vi "Measure Base.vi"(0 "eye scan in":refnum<class "niHighSpeedSerial Eye Scan v1 Host.lvclass">, 5 "requested number of new points":i32, 7 "timeout (100 ms)":dbl, 11 "error in":errorcluster) -> (4 "eye scan out":refnum<class "niHighSpeedSerial Eye Scan v1 Host.lvclass">, 6 "retrieved number of new points":i32, 8 "last point measured?":bool, 10 "timed out?":bool, 15 "error out":errorcluster)   [LabVIEW 2014, in "niHighSpeedSerial Eye Scan v1 Host.lvclass"]
doc: "The base Measure VI used by the various Measure VIs. This VI does the actual measurement, while the calling VIs do the data formatting.\n\n<B>Input Parameters</B>\n\n<B>eye scan in</B> Takes in a reference to your session from the previous VI.\n\n<B>requested number of new points</B> The number of new points to return, assuming that timeout is not reached, the entire scan doesn't complete, and no errors occur.\n\n<B>timeout (100 ms)</B> The amount of time (in seconds) before timing timing out.\nSpecifying '-1' prevents 'timed out' from ever returning true.\n\n<B>error in</B> describes error conditions that occur before this node runs. This input provides standard 'error in' functionality.\n\n<B>Output Parameters</B>\n\n<B>eye scan out</B> passes a reference to your session to the next VI.\n\n<B>retrieved number of new points</B> The number of new points that were retrieved in this call to Measure.\n\n<B>last point measured?</B> returns true if Eye Scan has completed measuring all points that it was configured to measure.\n\n<B>timed out?</B> returns true if at least 'timeout' amount of time has passed.\n\n<B>error out</B> contains error information. This output provides standard 'error out' functionality."
uses:
  <instrlib>/niHighSpeedSerial/Eye Scan/v1/Host/Eye Scan/niHighSpeedSerial Eye Scan v1 Host.lvclass
  <instrlib>/niHighSpeedSerial/Eye Scan/v1/Host/Eye Scan/niHighSpeedSerial Eye Scan v1 Host.lvclass/niHighSpeedSerial Eye Scan v1 Host.ctl
  <vilib>/Utility/error.llb/Error Cluster From Error Code.vi
  <vilib>/ErrorRing/Error Ring.xnode
  <instrlib>/niHighSpeedSerial/Eye Scan/v1/Host/Common/niHighSpeedSerial Eye Scan Common v1 Host.lvlib
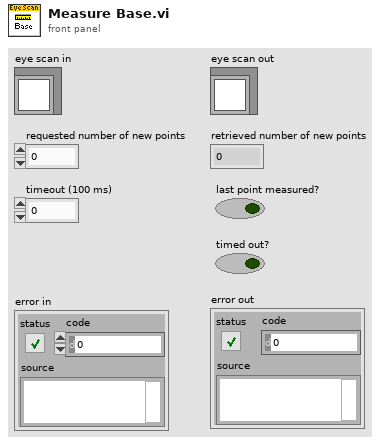
[diagram p1: front panel]
types:
  T1 = typedef "niHighSpeedSerial Eye Scan v1 Host.lvclass/Private Data.ctl" = cluster{"instruction target":refnum<class "niInstr Instruction Target v1 Host.lvclass">, "channels":T2[], "measure state":T3, "rx output divider":T4, "equalization mode":T5, "rx data width":T6, "BER floor":dbl, "number of points completed":i32, "rx output divider configured?":bool, "equalization mode configured?":bool, "rx data width configured?":bool}
  T2 = typedef "niHighSpeedSerial Eye Scan v1 Host.lvclass/Channel Data.ctl" = cluster{"instance":u8, "channel":refnum<class "niHighSpeedSerial Eye Scan Single Point v1 Host.lvclass">, "point iterator":refnum<class "niHighSpeedSerial Eye Scan Point Iterator v1 Host.lvclass">}
  T3 = typedef "niHighSpeedSerial Eye Scan v1 Host.lvclass/Measure State.ctl" = enum16{"Uninitialized", "Initialized", "Ready", "Measuring", "Finished", "Aborted"}
  T4 = typedef "niHighSpeedSerial Eye Scan Common v1 Host.lvlib/RX Output Divider.ctl" = enum16{"1", "2", "4", "8", "16"}
  T5 = typedef "niHighSpeedSerial Eye Scan Common v1 Host.lvlib/Equalization Mode.ctl" = enum16{"DFE", "LPM"}
  T6 = typedef "niHighSpeedSerial Eye Scan Common v1 Host.lvlib/Data Width.ctl" = enum16{"16 Bit", "20 Bit", "32 Bit", "40 Bit"}
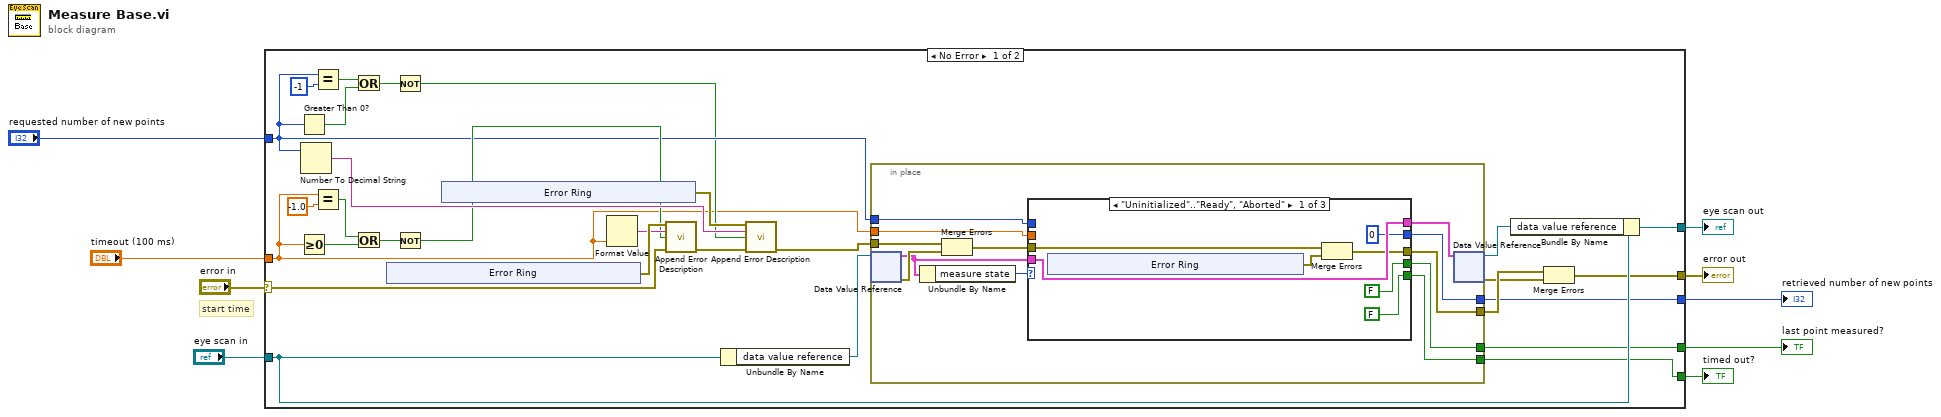
[diagram p0: block diagram]
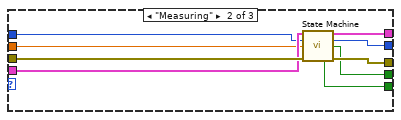
[diagram p2: hidden frame]
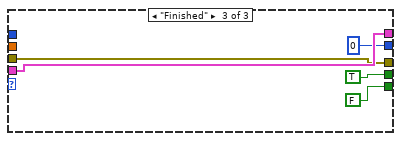
[diagram p3: hidden frame]
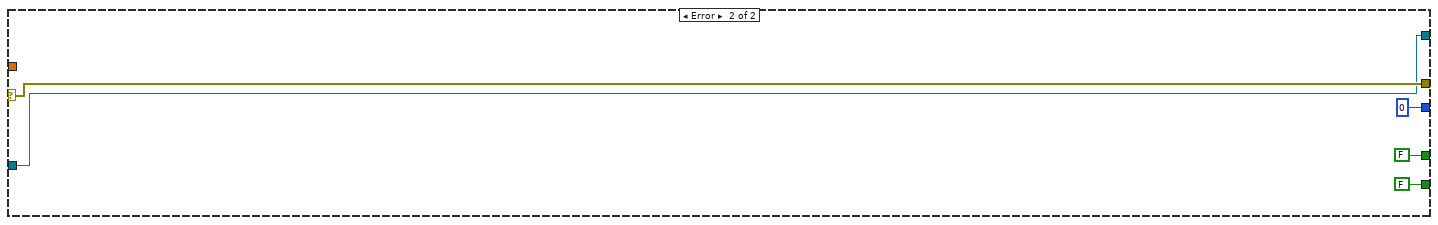
[diagram p4: hidden frame]
diagram:
  # "start time"
  n1 = case shown="No Error" "error in" {
    selector: "error in" -> [w28 w88]
    tunnel: [w32 w88] -> w8
    tunnel: [w37 w87] -> w7
    tunnel: "eye scan in" -> [w36 w87]
    tunnel: [w30 FALSE ("Last Point Measured?")] -> w5
    tunnel: [w29 FALSE ("Last Point Measured?")] -> w4
    tunnel: [w31 0 ("Retrieved Number of New Points")] -> w3
    tunnel: "requested number of new points" -> [w13 _]
    tunnel: "timeout (100 ms)" -> [w10 _]
    frame No Error {
      n2 = Greater Than 0?(x=w13) -> (x > 0?=w14:bool)
      n3 = Greater Or Equal To 0?(x=w10) -> (x >= 0?=w20:bool)
      n4 = Number To Decimal String(number=w13) -> (decimal integer string=w24:string)  [unwired: 1 in]
      n5 = Equal?(x=w13, y=-1) -> (x = y?=w15:bool)
      n6 = Equal?(x=w10, y=-1.0) -> (x = y?=w19:bool)
      n7 = Or(x=w15, y=w14) -> (x .or. y?=w16:bool)
      n8 = Or(x=w19, y=w20) -> (x .or. y?=w18:bool)
      n9 = xnode "Error Ring"() -> ("error out"=w27:errorcluster)
      n10 = Not(x=w16) -> (.not. x?=w11:bool)
      n11 = Not(x=w18) -> (.not. x?=w17:bool)
      n12 = xnode "Error Ring"() -> ("error out"=w22:errorcluster)
      n13 = Format Value(value (0)=w10) -> (output string=w26:string)  [unwired: 2 in]
      n14 = call <instrlib>:"Append Error Description.vi"("error to append"=w27, "append string (\"\")"=w26, "generate error?"=w17, "error in"=w28) -> ("error out"=w25:errorcluster)  [unwired: 11 in]
      n15 = Unbundle By Name(w36) -> ("data value reference"=w38:refnum<data-value>)
      n16 = call <instrlib>:"Append Error Description.vi"("error to append"=w22, "append string (\"\")"=w24, "generate error?"=w11, "error in"=w25) -> ("error out"=w23:errorcluster)  [unwired: 11 in]
      n17 = in-place {
        in-place-border: w23 -> [w58]
        in-place-border: [w54] -> w34
        in-place-border: [w51] -> w31
        in-place-border: w13 -> [w50]
        in-place-border: w10 -> [w49]
        in-place-border: [w48] -> w30
        in-place-border: [w47] -> w29
        n18 = in-place-dvr #1(w38) -> (w53:T1, w57:errorcluster)
        n19 = Unbundle By Name(w53) -> ("measure state"=w56:T3)
        n20 = Merge Errors(w58, w57) -> (w55:errorcluster)
        n21 = case shown="\"Uninitialized\"..\"Ready\", \"Aborted\"" w56 {
          tunnel: w55 -> [w63 w78 w81]
          tunnel: [w64 w77 w81] -> w54
          tunnel: w53 -> [w65 w76 w83]
          tunnel: [w65 w75 w83] -> w52
          tunnel: [0 ("Retrieved Number of New Points") w74 0 ("Retrieved Number of New Points")] -> w51
          tunnel: w50 -> [_ w73 _]
          tunnel: w49 -> [_ w72 _]
          tunnel: [FALSE ("Last Point Measured") w71 TRUE ("Last Point Measured")] -> w48
          tunnel: [FALSE ("Timed out?") w70 FALSE ("Timed out?")] -> w47
          frame "Uninitialized".."Ready", "Aborted" {
            n22 = xnode "Error Ring"() -> ("error out"=w59:errorcluster)
            n23 = Merge Errors(w63, w59) -> (w64:errorcluster)
          }
          frame "Measuring" {
            n24 = call <instrlib>:"State Machine.vi"("private data"=w76, "requested number of new points"=w73, "timeout (100 ms)"=w72, "error in"=w78) -> ("private data out"=w75:T1, "retrieved number of new points"=w74:i32, "last point measured?"=w71:bool, "timed out?"=w70:bool, "error out"=w77:errorcluster)  [unwired: 7 in]
          }
          frame "Finished" {
          }
        }
        n25 = in-place-dvr #1(w52) -> (w35:refnum<data-value>, w33:errorcluster)
      }
      n26 = Bundle By Name(cluster=w36, "data value reference"=w35) -> (w37:refnum<class "niHighSpeedSerial Eye Scan v1 Host.lvclass">)
      n27 = Merge Errors(w34, w33) -> (w32:errorcluster)
    }
    frame Error {
    }
  }
  "last point measured?" <- w5
  "retrieved number of new points" <- w3
  "eye scan out" <- w7
  "error out" <- w8
  "timed out?" <- w4
